vi "FTIR_Dialog_ScreenShots.vi"(8 "error in":errorcluster, 11 "Screenshots Pfad":path) -> (0 "error out":errorcluster, 3 "Screenshots Pfad  out":path caption="Screenshots Pfad")   [LabVIEW 2020, in "Backup.lvlib"]
uses:
  Backup.lvlib
  Seiten/FT-IR/Get Spectra/Get Spectra.lvlib
  Allgemein/allgemeine Sub-VIs.lvlib
  Seiten/FT-IR/Get Spectra/FTIR Diag.ctl
panel:
  in  "FTIR Diag":T1=1 items=["Background Igram", "Background sBeam", "sample Igram", "sample Background", "sample Absorbance"]
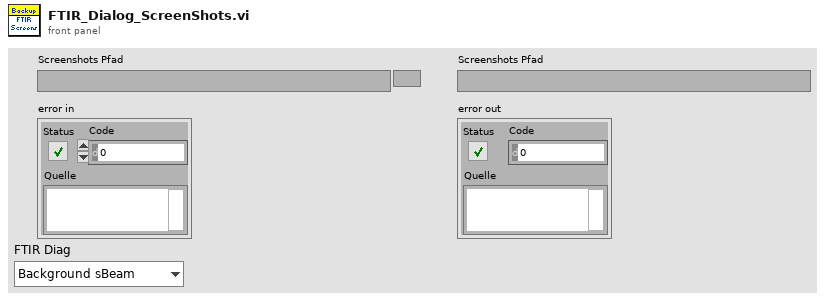
[diagram p1: front panel]
types:
  T1 = typedef "FT-IR.lvlib/Get Spectra.lvlib/FTIR Diag.ctl" = u16
  T2 = enum32{"Bad", "Idle", "Run top level", "Running"}
  T3 = typedef "imagedata.ctl" = cluster{"image type":i32, "image depth":i32, "image":u8[], "mask":u8[], "colors":u32[], "Rectangle":cluster{"left":i16, "top":i16, "right":i16, "bottom":i16}}
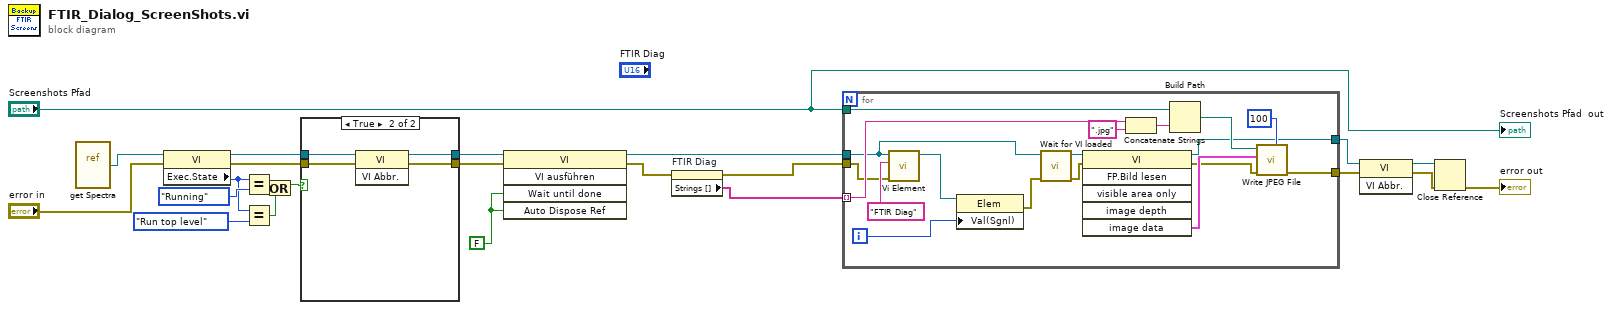
[diagram p0: block diagram]
diagram:
  w14 = FALSE
  n1 = vi-ref "get Spectra.vi"() -> (w17:refnum<vi>)
  n2 = property class="VI"(reference=w17, error in="error in") -> (reference out=w13:refnum<vi>, error out=w10:errorcluster, "Exec.State"=w7:T2)
  n3 = Equal?(x=w7, y=T2."Running" ("Ausführung:Status")) -> (x = y?=w11:bool)
  n4 = Equal?(x=w7, y=T2."Run top level" ("Ausführung:Status")) -> (x = y?=w5:bool)
  n5 = Or(x=w11, y=w5) -> (x .or. y?=w6:bool)
  n6 = case shown="True" w6 {
    tunnel: w13 -> [w25 w29]
    tunnel: [w25 w28] -> w12
    tunnel: w10 -> [w24 w27]
    tunnel: [w24 w26] -> w9
    frame False {
    }
    frame True {
      n7 = invoke class="VI" method="VI Abbr."(reference=w29, error in=w27) -> (reference out=w28:refnum<vi>, error out=w26:errorcluster)  [unwired: 1 in, 1 out]
    }
  }
  n8 = invoke class="VI" method="VI ausführen"(reference=w12, error in=w9, "Wait until done"=w14, "Auto Dispose Ref"=w14) -> (reference out=w23:refnum<vi>, error out=w2:errorcluster)  [unwired: 1 in, 3 out]
  n9 = property on="FTIR Diag" class="Ring (strikt)"(error in=w2) -> (error out=w1:errorcluster, "Strings []"=w3:string[])  [unwired: 1 in, 1 out]
  n10 = for {
    tunnel: w3 -> [w40] mode=indexing
    tunnel: w1 -> [w34]
    tunnel: "Screenshots Pfad" -> [w41]
    tunnel: [w39] -> w22
    tunnel: w23 -> [w30]
    tunnel: [w38] -> w21
    i -> [w32]
    n11 = call "Vi Element.vi"("Fehler (in)"=w34, "Element Beschriftiung"="FTIR Diag" ("Elementname"), "VI Referenz"=w30) -> ("Elem Referenz"=w33:refnum<vi>)  [unwired: 7 in, 1 out]
    n12 = property class="Elem"(reference=w33, "Val(Sgnl)"=w32) -> (error out=w31:errorcluster)  [unwired: 1 in, 1 out]
    n13 = call "Wait for VI loaded.vi"("error in"=w31, "VI Referenz"=w30) -> ("error out"=w36:errorcluster, "VI Referenz out"=w37:refnum<vi>)  [unwired: 7 in, 1 out]
    n14 = invoke class="VI" method="FP.Bild lesen"(reference=w37, error in=w36) -> (reference out=w38:refnum<vi>, error out=w46:errorcluster, "image data"=w47:T3)  [unwired: 4 in, 3 out]
    n15 = Concatenate Strings(w40, ".jpg" ("String")) -> (w43:string)
    n16 = Build Path(base path=w41, name or relative path=w43) -> (appended path=w44:path)
    n17 = call <vilib>:"Write JPEG File.vi"("quality (80)"=100, "error in (no error)"=w46, "image data"=w47, "path to JPEG file"=w44) -> ("error out"=w39:errorcluster)  [unwired: 6 in, 1 out]
  }
  n18 = invoke class="VI" method="VI Abbr."(reference=w21, error in=w22) -> (reference out=w20:refnum<vi>, error out=w19:errorcluster)  [unwired: 1 in, 1 out]
  n19 = Close Reference(reference=w20, error in (no error)=w19) -> (error out=→"error out":errorcluster)
  "Screenshots Pfad  out" <- "Screenshots Pfad"
